vi "2-10.vi"() -> ()   [LabVIEW 2022 SP3]
panel:
  in  "年龄":u8
  in  "姓名":string
  in  "学号":string
  out "学生记录":cluster{"学号串":string, "姓名":string, "数值":dbl}
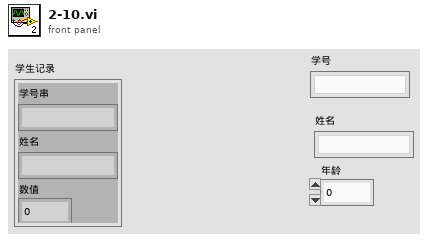
[diagram p1: front panel]
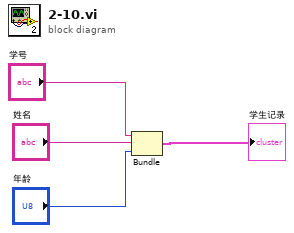
[diagram p0: block diagram]
diagram:
  n1 = Bundle("学号"="学号", "姓名"="姓名", "年龄"="年龄") -> (→"学生记录":cluster{"学号":string, "姓名":string, "年龄":u8})  [unwired: 1 in]
